vi "Build ADU.vi"(8 "error in (no error)":errorcluster, 10 "Slave ID":u8, 11 "MB_ADU in":refnum<class "MB_ADU.lvclass">) -> (0 "error out":errorcluster, 3 "MB_ADU out":refnum<class "MB_ADU.lvclass">)   [LabVIEW 2023, in "Jiaxin_Stepper_Controller.lvlib" / "MB Master.lvlib" / "MB_ADU.lvclass"]
doc: "Build the ADU for a Modbus master over serial line.\n\nThis sets the slave address and resets the RX and TX timestamps."
uses:
  MB_ADU.lvclass
  MB_ADU.lvclass/MB_ADU.ctl
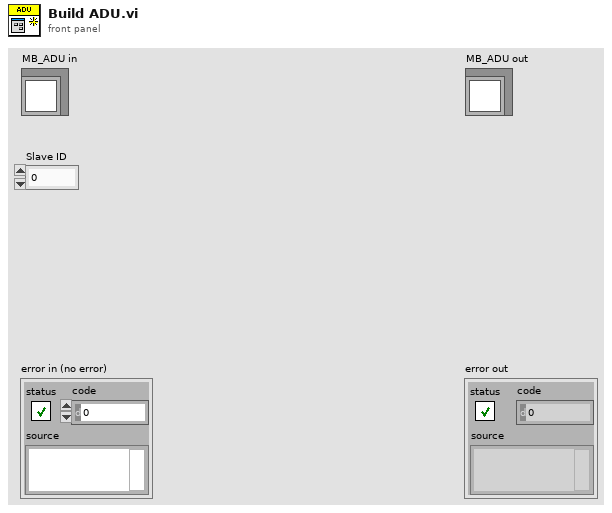
[diagram p1: front panel]
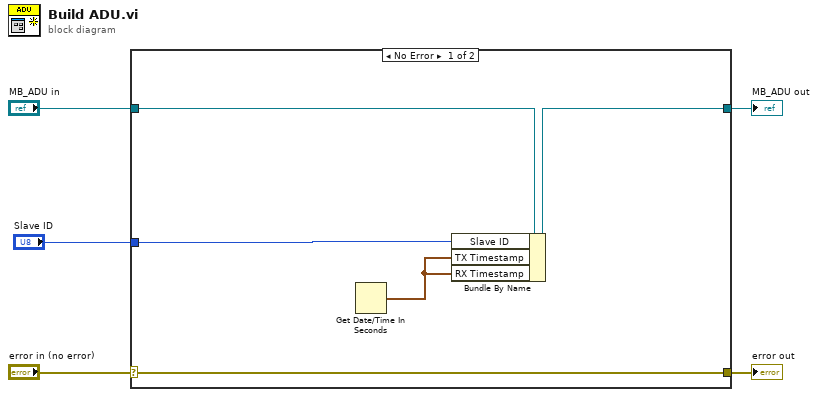
[diagram p0: block diagram]
diagram:
  n1 = case shown="No Error" "error in (no error)" {
    selector: "error in (no error)" -> [w10 w12]
    tunnel: [w10 w12] -> w4
    tunnel: [w8 w11] -> w2
    tunnel: "MB_ADU in" -> [w9 w11]
    tunnel: "Slave ID" -> [w7 _]
    frame No Error {
      n2 = Get Date/Time In Seconds() -> (seconds since 1Jan1904=w6:timestamp)
      n3 = Bundle By Name(cluster=w9, "Slave ID"=w7, "TX Timestamp"=w6, "RX Timestamp"=w6) -> (w8:refnum<class "MB_ADU.lvclass">)
    }
    frame Error {
    }
  }
  "error out" <- w4
  "MB_ADU out" <- w2
